vi "用Case结构处理错误.vi"() -> ()   [LabVIEW 2010]
uses:
  Instance           2 26Saved   用Case结构处理错误 .vi
  Instance           4 26Saved   用Case结构处理错误 .vi
  Instance           3 26Saved   用Case结构处理错误 .vi
  Instance           1 26Saved   用Case结构处理错误 .vi
panel:
  out "信号算术平均值":dbl
  out "信号状态":string
  out "信号状态":string
  out "信号算术平均值":dbl
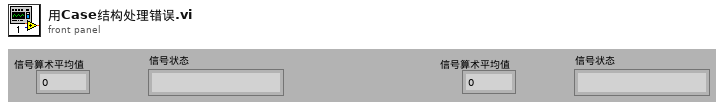
[diagram p1: front panel]
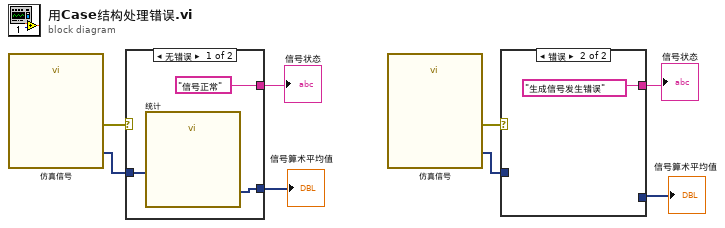
[diagram p0: block diagram]
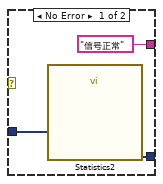
[diagram p2: hidden frame]
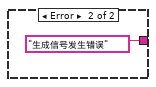
[diagram p3: hidden frame]
diagram:
  n1 = call "仿真信号"() -> ("正弦与均匀噪声"=w7:dynamicdata, "error out"=w8:errorcluster)  [unwired: 14 in]
  n2 = case shown="无错误" w8 {
    tunnel: w7 -> [w11 _]
    tunnel: [w9 _] -> w6
    tunnel: ["信号正常" "生成信号发生错误"] -> w5
    frame No Error {
      n3 = call "统计"("Signals"=w11) -> ("Arithmetic Mean"=w9:dynamicdata)  [unwired: 25 in, 1 out]
    }
    frame Error {
    }
  }
  "信号算术平均值" <- w6
  "信号状态" <- w5
  n4 = call "仿真信号"() -> ("正弦与均匀噪声"=w2:dynamicdata, "error out"=w1:errorcluster)  [unwired: 14 in]
  n5 = case shown="错误" w1 {
    tunnel: w2 -> [w15 _]
    tunnel: [w14 _] -> w3
    tunnel: ["信号正常" "生成信号发生错误"] -> w4
    frame No Error {
      n6 = call "Statistics2"("Signals"=w15) -> ("Arithmetic Mean"=w14:dynamicdata)  [unwired: 25 in, 1 out]
    }
    frame Error {
    }
  }
  "信号算术平均值" <- w3
  "信号状态" <- w4
